vi "QuadAnalyzer.vi"() -> ()   [LabVIEW 2012]
uses:
  <instrlib>/niScope/Controls/niScope trigger source.ctl
  <instrlib>/niScope/Controls/niScope vertical coupling.ctl
  <instrlib>/niScope/Configure/Trigger/niScope Configure Trigger Edge.vi
  <instrlib>/niScope/Acquire/Fetch/niScope Multi Fetch Cluster.vi
  <vilib>/Analysis/baseanly.llb/Mean (DBL).vi
  <vilib>/Analysis/NI_AALBase.lvlib
panel:
  in  "Signal Source 2":T1="3" caption="Y Signal Source"
  in  "Signal Coupling":T2=1 caption="vertical coupling" items=["AC", "DC", "Ground"]
  in  "Signal Source":T1="1" caption="X Signal Source"
  in  "Reference Position (%)":dbl=10.0 caption="Reference Position" format="%.1f"
  out "Total Acquisition Time (s)":dbl
  out "Scope Traces":dynamicdata(graph)
  in  "min sample rate":dbl=10000.0 caption="Sample Rate (Max 20M)" format="%^.2e"
  in  "Trigger Level":dbl=2.0 format="%.2f"
  in  "Trigger Source":T1="0"
  in  "Number of Records":i32=30000 caption="Number of Samples"
  # "Settings can be modified \nin real-time (updates every 10s or so)."
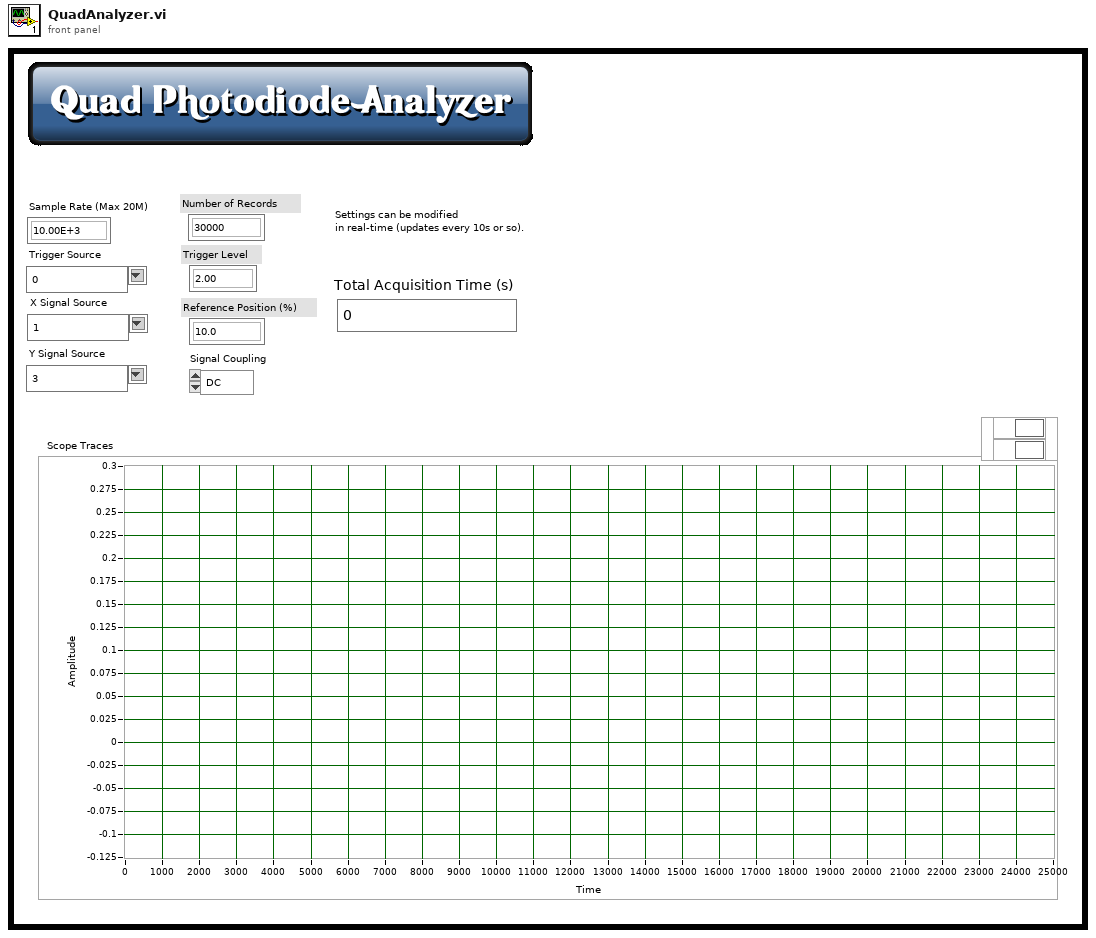
[diagram p1: front panel]
types:
  T1 = typedef "niScope trigger source.ctl" = string
  T2 = typedef "niScope vertical coupling.ctl" = i32
  T3 = cluster{"relativeInitialX":dbl, "xIncrement":dbl, "wfm":dbl[]}[]
  T4 = cluster{"relativeInitialX":dbl, "xIncrement":dbl, "wfm":dbl[]}
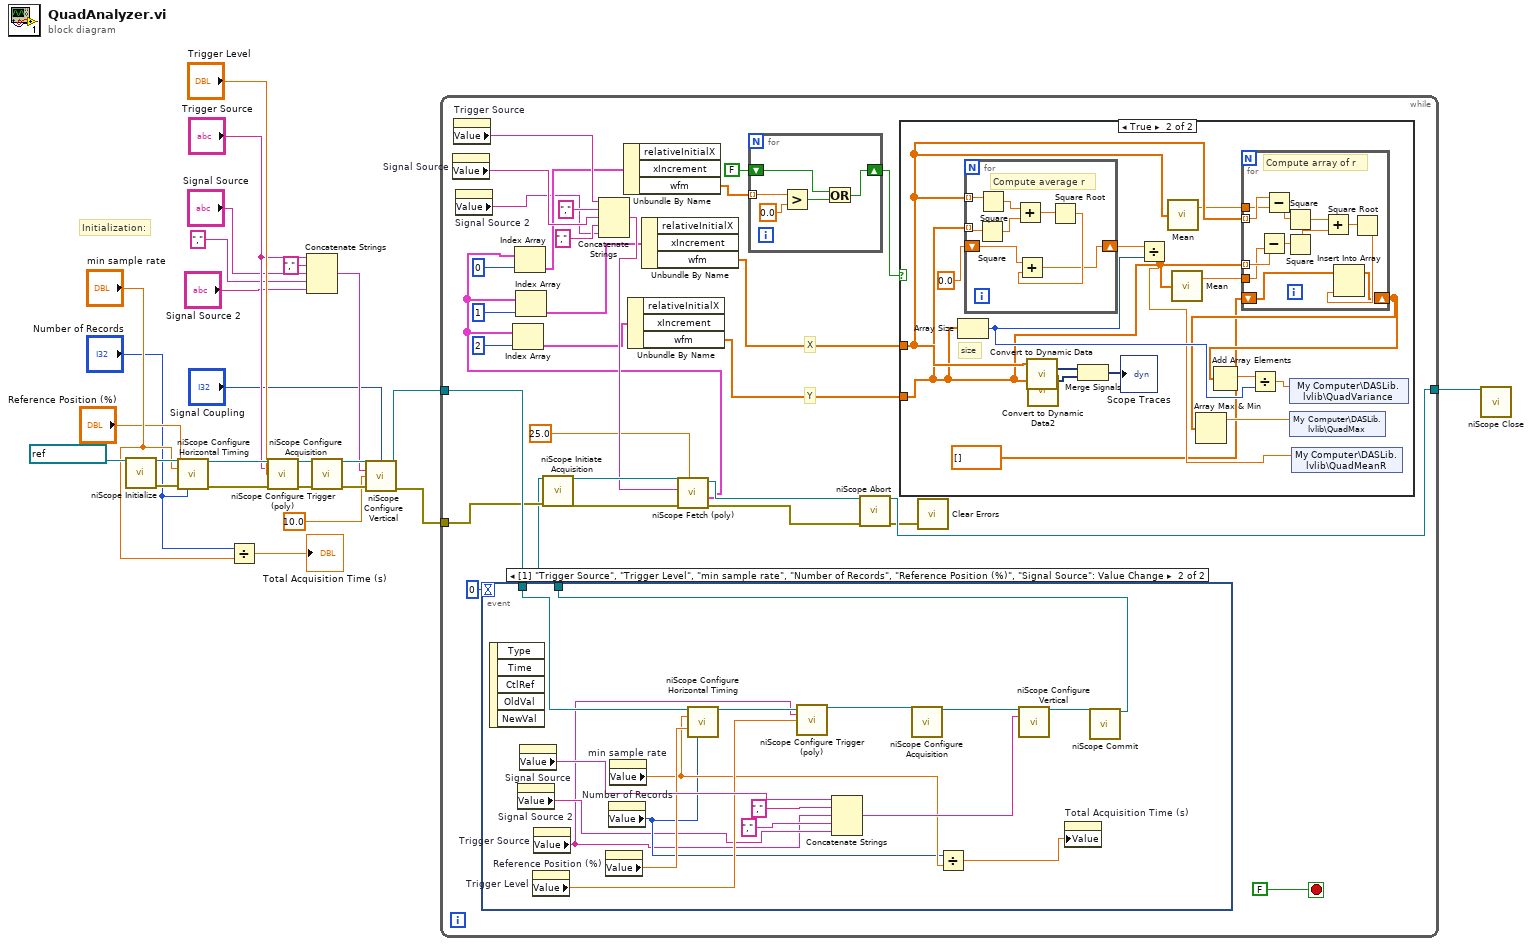
[diagram p0: block diagram]
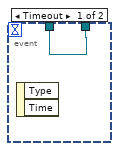
[diagram p2: hidden frame]
diagram:
  # "Initialization:"
  n1 = call <instrlib>:"niScope Initialize.vi"("resource name"=refnum<k15> "PXI1Slot4") -> ("instrument handle"=w24:refnum<k15>, "error out"=w23:errorcluster)  [unwired: 13 in]
  n2 = call <instrlib>:"niScope Configure Horizontal Timing.vi"("instrument handle"=w24, "min sample rate"="min sample rate", "reference position"="Reference Position (%)", "error in"=w23, "min record length"="Number of Records") -> ("instrument handle out"=w22:refnum<k15>, "error out"=w13:errorcluster)  [unwired: 9 in]
  n3 = Divide(x="Number of Records", y="min sample rate") -> (x/y=→"Total Acquisition Time (s)":dbl)
  n4 = call-poly <instrlib>:"niScope Configure Trigger (poly).vi"("instrument handle"=w22, "trigger source"="Trigger Source", "trigger level"="Trigger Level", "error in"=w13) -> ("instrument handle out"=w19:refnum<k15>, "error out"=w18:errorcluster)  [unwired: 10 in]
  n5 = Concatenate Strings("Trigger Source", "," ("string"), "Signal Source", "," ("string"), "Signal Source 2") -> (w7:string)
  n6 = call <instrlib>:"niScope Configure Acquisition.vi"("instrument handle"=w19, "error in"=w18) -> ("instrument handle out"=w16:refnum<k15>, "error out"=w17:errorcluster)  [unwired: 12 in]
  n7 = call <instrlib>:"niScope Configure Vertical.vi"("instrument handle"=w16, "vertical coupling"="Signal Coupling", "channels"=w7, "vertical range"=10.0, "error in"=w17) -> ("instrument handle out"=w20:refnum<k15>, "error out"=w15:errorcluster)  [unwired: 9 in]
  n8 = while {
    tunnel: w20 -> [w47]
    tunnel: w15 -> [w46]
    tunnel: [w54] -> w14
    stop <- FALSE ("stop") stop-if-true
    # "Y"
    # "X"
    n9 = property on="Signal Source" class="CmbBox (strict)"() -> ("Value"=w42:T1)  [unwired: 2 in, 2 out]
    n10 = property on="Trigger Source" class="CmbBox (strict)"() -> ("Value"=w44:T1)  [unwired: 2 in, 2 out]
    n11 = property on="Signal Source 2" class="CmbBox (strict)"() -> ("Value"=w31:T1)  [unwired: 2 in, 2 out]
    n12 = event shown="[1] \"Trigger Source\", \"Trigger Level\", \"min sample rate\", \"Number of Records\", \"Reference Position (%)\", \"Signal Source\": Value Change" {
      selector: _ -> [_ _]
      dyn-events: _ -> [_ _]
      timeout: 0 -> [_ _]
      tunnel: w47 -> [w56 w73]
      tunnel: [w56 w62] -> w35
      event Timeout {
        n13 = event-data() -> ()  [unwired: 1 in, 2 out]
      }
      event "Trigger Level", "min sample rate", "Number of Records", "Reference Position (%)": Value Change {
        n14 = event-data() -> ()  [unwired: 1 in, 5 out]
        n15 = property on="Signal Source 2" class="CmbBox (strict)"() -> ("Value"=w58:T1)  [unwired: 2 in, 2 out]
        n16 = property on="Signal Source" class="CmbBox (strict)"() -> ("Value"=w67:T1)  [unwired: 2 in, 2 out]
        n17 = property on="Trigger Level" class="DigNum (strict)"() -> ("Value"=w65:dbl)  [unwired: 2 in, 2 out]
        n18 = property on="Trigger Source" class="CmbBox (strict)"() -> ("Value"=w57:T1)  [unwired: 2 in, 2 out]
        n19 = property on="Reference Position (%)" class="DigNum (strict)"() -> ("Value"=w66:dbl)  [unwired: 2 in, 2 out]
        n20 = property on="Number of Records" class="DigNum (strict)"() -> ("Value"=w61:i32)  [unwired: 2 in, 2 out]
        n21 = property on="min sample rate" class="DigNum (strict)"() -> ("Value"=w64:dbl)  [unwired: 2 in, 2 out]
        n22 = call <instrlib>:"niScope Configure Horizontal Timing.vi"("instrument handle"=w73, "min sample rate"=w64, "reference position"=w66, "min record length"=w61) -> ("instrument handle out"=w72:refnum<k15>)  [unwired: 10 in, 1 out]
        n23 = call-poly <instrlib>:"niScope Configure Trigger (poly).vi"("instrument handle"=w72, "trigger source"=w57, "trigger level"=w65) -> ("instrument handle out"=w71:refnum<k15>)  [unwired: 11 in, 1 out]
        n24 = Concatenate Strings(w67, "," ("string"), w57, "," ("string"), w58) -> (w69:string)
        n25 = call <instrlib>:"niScope Configure Acquisition.vi"("instrument handle"=w71) -> ("instrument handle out"=w70:refnum<k15>)  [unwired: 13 in, 1 out]
        n26 = Divide(x=w61, y=w64) -> (x/y=w60:dbl)
        n27 = call <instrlib>:"niScope Configure Vertical.vi"("instrument handle"=w70, "channels"=w69) -> ("instrument handle out"=w63:refnum<k15>)  [unwired: 12 in, 1 out]
        n28 = property on="Total Acquisition Time (s)" class="DigNum (strict)"("Value"=w60) -> ()  [unwired: 2 in, 2 out]
        n29 = call <instrlib>:"niScope Commit.vi"("instrument handle"=w63) -> ("instrument handle out"=w62:refnum<k15>)  [unwired: 13 in, 1 out]
      }
    }
    n30 = call <instrlib>:"niScope Initiate Acquisition.vi"("instrument handle"=w35, "error in"=w46) -> ("instrument handle out"=w45:refnum<k15>, "error out"=w40:errorcluster)  [unwired: 12 in]
    n31 = Concatenate Strings(w44, "," ("string"), w42, "," ("string"), w31) -> (w41:string)
    n32 = call-poly <instrlib>:"niScope Fetch (poly).vi"("timeout"=25.0, "error in"=w40, "channels"=w41, "instrument handle"=w45) -> ("error out"=w39:errorcluster, "waveform"=w29:T3, "instrument handle out"=w38:refnum<k15>)  [unwired: 4 in, 1 out]
    n33 = Index Array(array=w29, index=2) -> (element=w28:T4)
    n34 = Index Array(array=w29, index=0) -> (element=w37:T4)
    n35 = Index Array(array=w29, index=1) -> (element=w36:T4)
    n36 = Unbundle By Name(w37) -> ("wfm"=w34:dbl[])  [unwired: 2 out]
    n37 = Unbundle By Name(w28) -> ("wfm"=w27:dbl[])  [unwired: 2 out]
    n38 = Unbundle By Name(w36) -> ("wfm"=w33:dbl[])  [unwired: 2 out]
    n39 = for {
      tunnel: w34 -> [w74] mode=indexing
      shift-right: [w75] -> w50
      shift-left: FALSE -> [w76]
      n40 = Greater?(x=w74, y=0.0) -> (0:w77:bool)
      n41 = Or(x=w76, y=w77) -> (x .or. y?=w75:bool)
    }
    n42 = call <instrlib>:"niScope Abort.vi"("instrument handle"=w38, "error in"=w39) -> ("instrument handle out"=w54:refnum<k15>, "error out"=w53:errorcluster)  [unwired: 12 in]
    n43 = case shown="True" w50 {
      tunnel: w33 -> [_ w84]
      tunnel: w27 -> [_ w83]
      frame False {
      }
      frame True {
        # "size"
        n44 = Array Size(array=w83) -> (size(s)=w88:i32)
        n45 = for {
          tunnel: w84 -> [w114] mode=indexing
          tunnel: w83 -> [w113] mode=indexing
          shift-right: [w107] -> w91
          shift-left: 0.0 -> [w109]
          # "Compute average r"
          n46 = Square(x=w113) -> (x^2=w111:dbl)
          n47 = Square(x=w114) -> (x^2=w112:dbl)
          n48 = Add(x=w112, y=w111) -> (x+y=w110:dbl)
          n49 = Square Root(x=w110) -> (sqrt(x)=w108:dbl)
          n50 = Add(x=w109, y=w108) -> (x+y=w107:dbl)
        }
        n51 = call "Convert to Dynamic Data"("Array"=w84) -> ("Dynamic Data Type"=w94:dynamicdata)  [unwired: 3 in]
        n52 = call "Convert to Dynamic Data2"("Array"=w83) -> ("Dynamic Data Type"=w93:dynamicdata)  [unwired: 3 in]
        n53 = Merge Signals(w94, w93) -> (→"Scope Traces":dynamicdata)
        n54 = Divide(x=w91, y=w88) -> (x/y=w80:dbl)
        n55 = call-poly <vilib>:"Mean.vi"("X"=w84) -> ("mean"=w82:dbl)  [unwired: 1 out]
        n56 = call-poly <vilib>:"Mean.vi"("X"=w83) -> ("mean"=w81:dbl)  [unwired: 1 out]
        n57 = for {
          tunnel: w84 -> [w99] mode=indexing
          tunnel: w83 -> [w101] mode=indexing
          shift-right: [w95] -> w87
          shift-left: dbl[] [] -> [w106]
          tunnel: w82 -> [w98]
          tunnel: w81 -> [w100]
          # "Compute array of r"
          n58 = Subtract(x=w101, y=w100) -> (x-y=w104:dbl)
          n59 = Subtract(x=w99, y=w98) -> (x-y=w105:dbl)
          n60 = Square(x=w105) -> (x^2=w97:dbl)
          n61 = Square(x=w104) -> (x^2=w96:dbl)
          n62 = Add(x=w97, y=w96) -> (x+y=w103:dbl)
          n63 = Square Root(x=w103) -> (sqrt(x)=w102:dbl)
          n64 = Insert Into Array(array=w106, new element=w102) -> (w95:dbl[])  [unwired: 1 in]
        }
        n65 = Array Max & Min(array=w87) -> (max value=w85:dbl)  [unwired: 3 out]
        n66 = Add Array Elements(numeric array=w87) -> (sum=w89:dbl)
        n67 = Divide(x=w89, y=w88) -> (x/y=w86:dbl)
        n68 = shared-variable "My Computer\\DASLib.lvlib\\QuadVariance"(w86) -> ()  [unwired: 1 in, 1 out]
        n69 = shared-variable "My Computer\\DASLib.lvlib\\QuadMax"(w85) -> ()  [unwired: 1 in, 1 out]
        n70 = shared-variable "My Computer\\DASLib.lvlib\\QuadMeanR"(w80) -> ()  [unwired: 1 in, 1 out]
      }
    }
    n71 = call <vilib>:"Clear Errors.vi"("error in (no error)"=w53) -> ()  [unwired: 6 in, 1 out]
  }
  n72 = call <instrlib>:"niScope Close.vi"("instrument handle"=w14) -> ()  [unwired: 14 in, 1 out]
